vi "motor correction.vi"(0 "Rotate_angle":dbl, 4 "first or second":bool, 5 "last rotate angle":dbl, 6 "Encoder_Count":dbl=109958.0, 7 "Direction":T1(ring), 8 "Stand Position":T4, 9 "encoder position":T3={"Encoder Position 5"=-9, "Encoder Position 1"=20, "Encoder Position 0"=55402, "Encoder Position 2"=-7, "Encoder Position 7"=4, "Encoder Position 6"=-3}, 10 "set position 2":dbl, 11 "set position":dbl) -> (1 "current rotate angle":dbl, 2 "Setpoint_to_motor":T2)   [LabVIEW 2019]
panel:
  out "output":dbl(graph)
  out "input":dbl(graph)
  out "x < y?":bool
  out "last rotate angle 2":dbl
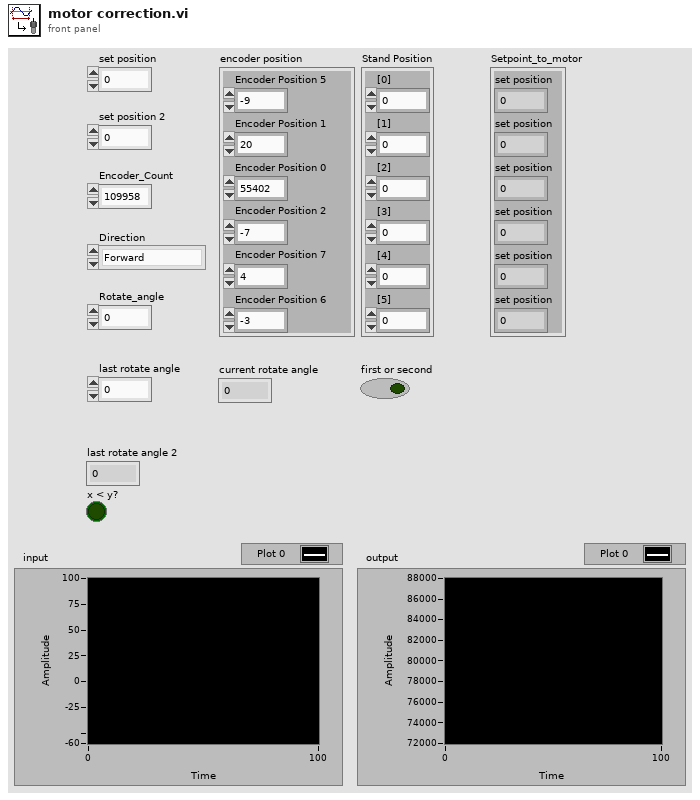
[diagram p1: front panel]
types:
  T1 = enum16{"Forward", "Left", "Right", "Forward+Left", "Forward+Right"}
  T2 = cluster{"set position":dbl, "set position":dbl, "set position":dbl, "set position":dbl, "set position":dbl, "set position":dbl}
  T3 = cluster{"Encoder Position 5":i32, "Encoder Position 1":i32, "Encoder Position 0":i32, "Encoder Position 2":i32, "Encoder Position 7":i32, "Encoder Position 6":i32}
  T4 = cluster{"[0]":dbl, "[1]":dbl, "[2]":dbl, "[3]":dbl, "[4]":dbl, "[5]":dbl}
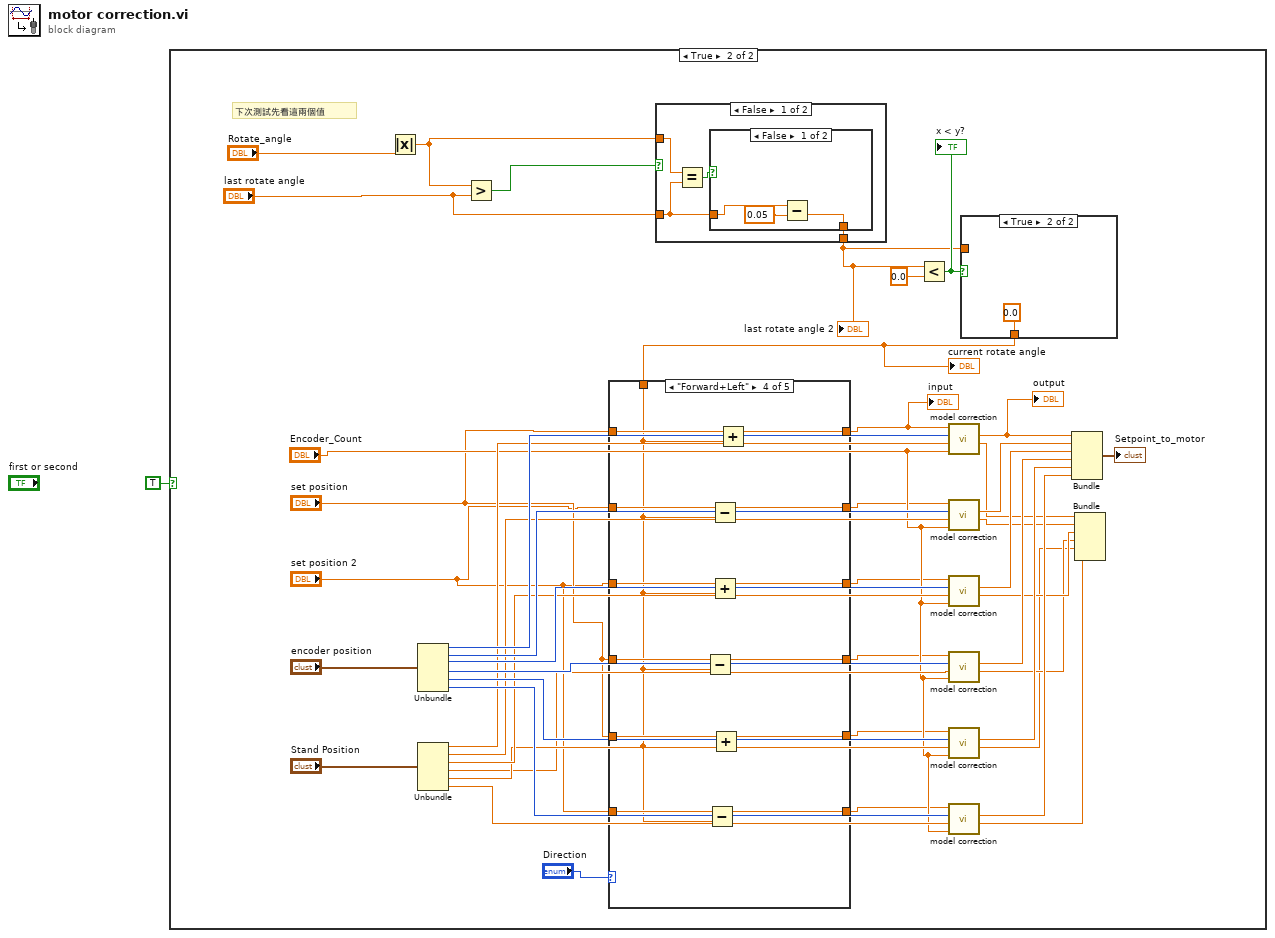
[diagram p0: block diagram]
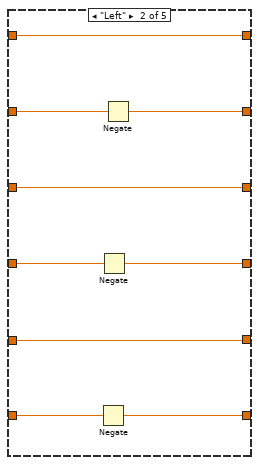
[diagram p4: hidden frame]
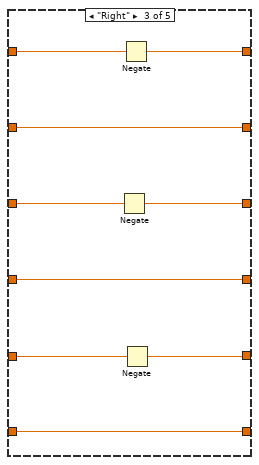
[diagram p5: hidden frame]
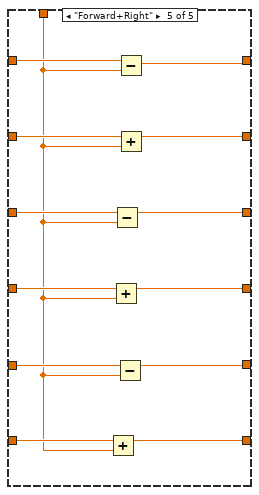
[diagram p6: hidden frame]
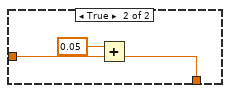
[diagram p9: hidden frame]
diagram:
  n1 = case shown="True" TRUE {
    frame False {
    }
    frame True {
      # "下次測試先看這兩個值"
      n2 = Absolute Value(x="Rotate_angle") -> (abs(x)=w20:dbl)
      n3 = Unbundle("encoder position") -> ("Encoder Position 5"=w44:i32, "Encoder Position 1"=w43:i32, "Encoder Position 0"=w42:i32, "Encoder Position 2"=w41:i32, "Encoder Position 7"=w40:i32, "Encoder Position 6"=w39:i32)
      n4 = Unbundle("Stand Position") -> ("[0]"=w38:dbl, "[1]"=w37:dbl, "[2]"=w36:dbl, "[3]"=w14:dbl, "[4]"=w35:dbl, "[5]"=w34:dbl)
      n5 = Greater?(x=w20, y="last rotate angle") -> (0:w21:bool)
      n6 = case shown="False" w21 {
        tunnel: "last rotate angle" -> [w100 w109]
        tunnel: [w99 w108] -> w17
        tunnel: w20 -> [w102 _]
        frame False {
          n7 = Equal?(x=w102, y=w100) -> (x = y?=w101:bool)
          n8 = case shown="False" w101 {
            tunnel: w100 -> [w104 w106]
            tunnel: [w105 w106] -> w99
            frame False {
              n9 = Subtract(x=w104, y=0.05 ("x")) -> (x-y=w105:dbl)
            }
            frame True {
            }
          }
        }
        frame True {
          n10 = Add(x=0.05, y=w109) -> (x+y=w108:dbl)
        }
      }
      "last rotate angle 2" <- w17
      n11 = Less?(x=w17, y=0.0) -> (x < y?=w19:bool)
      "x < y?" <- w19
      n12 = case shown="True" w19 {
        tunnel: [w97 0.0 ("last rotate angle")] -> w5
        tunnel: w17 -> [w97 _]
        frame False {
        }
        frame True {
        }
      }
      "current rotate angle" <- w5
      n13 = case shown="\"Forward+Left\"" "Direction" {
        tunnel: "set position" -> [w52 w61 w70 w83 w96]
        tunnel: [w52 w61 w64 w82 w90] -> w3
        tunnel: "set position 2" -> [w49 w60 w69 w81 w95]
        tunnel: [w49 w59 w69 w76 w89] -> w9
        tunnel: [w48 w58 w63 w75 w88] -> w8
        tunnel: "set position 2" -> [w48 w58 w68 w80 w94]
        tunnel: "set position" -> [w51 w57 w67 w79 w93]
        tunnel: [w51 w54 w67 w74 w87] -> w12
        tunnel: [w50 w56 w62 w73 w86] -> w10
        tunnel: "set position" -> [w50 w56 w66 w78 w92]
        tunnel: "set position 2" -> [w47 w55 w65 w77 w91]
        tunnel: [w47 w53 w65 w72 w85] -> w6
        tunnel: w5 -> [_ _ _ w71 w84]
        frame "Forward", Default {
        }
        frame "Left" {
          n14 = Negate(x=w55) -> (-x=w53:dbl)
          n15 = Negate(x=w57) -> (-x=w54:dbl)
          n16 = Negate(x=w60) -> (-x=w59:dbl)
        }
        frame "Right" {
          n17 = Negate(x=w68) -> (-x=w63:dbl)
          n18 = Negate(x=w70) -> (-x=w64:dbl)
          n19 = Negate(x=w66) -> (-x=w62:dbl)
        }
        frame "Forward+Left" {
          n20 = Subtract(x=w79, y=w71) -> (x-y=w74:dbl)
          n21 = Subtract(x=w77, y=w71) -> (x-y=w72:dbl)
          n22 = Subtract(x=w81, y=w71) -> (x-y=w76:dbl)
          n23 = Add(x=w80, y=w71) -> (x+y=w75:dbl)
          n24 = Add(x=w78, y=w71) -> (x+y=w73:dbl)
          n25 = Add(x=w83, y=w71) -> (x+y=w82:dbl)
        }
        frame "Forward+Right" {
          n26 = Add(x=w91, y=w84) -> (x+y=w85:dbl)
          n27 = Add(x=w93, y=w84) -> (x+y=w87:dbl)
          n28 = Subtract(x=w94, y=w84) -> (x-y=w88:dbl)
          n29 = Subtract(x=w92, y=w84) -> (x-y=w86:dbl)
          n30 = Subtract(x=w96, y=w84) -> (x-y=w90:dbl)
          n31 = Add(x=w95, y=w84) -> (x+y=w89:dbl)
        }
      }
      "input" <- w3
      n32 = call "model correction.vi"("encoder count"="Encoder_Count", "stand position"=w38, "encoder"=w44, "virtual position"=w3) -> ("encoder position(Deg)"=w27:dbl, "set position"=w2:dbl)  [unwired: 6 in]
      "output" <- w2
      n33 = call "model correction.vi"("encoder count"="Encoder_Count", "stand position"=w37, "encoder"=w43, "virtual position"=w9) -> ("encoder position(Deg)"=w26:dbl, "set position"=w33:dbl)  [unwired: 6 in]
      n34 = call "model correction.vi"("encoder count"="Encoder_Count", "stand position"=w36, "encoder"=w42, "virtual position"=w8) -> ("encoder position(Deg)"=w25:dbl, "set position"=w32:dbl)  [unwired: 6 in]
      n35 = call "model correction.vi"("encoder count"="Encoder_Count", "stand position"=w14, "encoder"=w41, "virtual position"=w12) -> ("encoder position(Deg)"=w24:dbl, "set position"=w31:dbl)  [unwired: 6 in]
      n36 = call "model correction.vi"("encoder count"="Encoder_Count", "stand position"=w35, "encoder"=w40, "virtual position"=w10) -> ("encoder position(Deg)"=w23:dbl, "set position"=w30:dbl)  [unwired: 6 in]
      n37 = call "model correction.vi"("encoder count"="Encoder_Count", "stand position"=w34, "encoder"=w39, "virtual position"=w6) -> ("encoder position(Deg)"=w22:dbl, "set position"=w29:dbl)  [unwired: 6 in]
      n38 = Bundle("set position"=w2, "set position"=w33, "set position"=w32, "set position"=w31, "set position"=w30, "set position"=w29) -> (→"Setpoint_to_motor":T2)  [unwired: 1 in]
      n39 = Bundle("encoder position(Deg)"=w27, "encoder position(Deg)"=w26, "encoder position(Deg)"=w25, "encoder position(Deg)"=w24, "encoder position(Deg)"=w23, "encoder position(Deg)"=w22) -> ()  [unwired: 1 in, 1 out]
    }
  }
